vi "Cache-Kill.vi"(8 "error in":errorcluster, 11 "Idx":i32) -> (0 "error out":errorcluster)   [LabVIEW 2016]
uses:
  Cache.Action.ctl
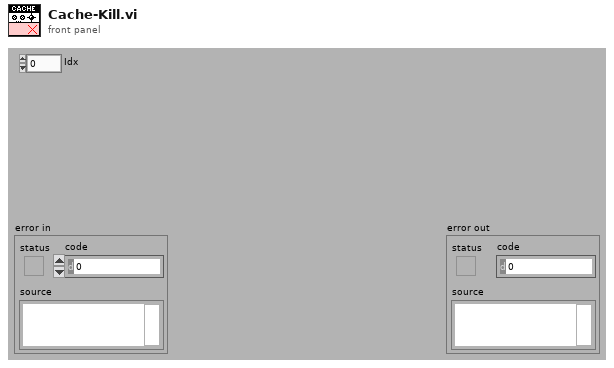
[diagram p1: front panel]
types:
  T1 = typedef "Cache.Action.ctl" = enum32{"idle", "constructor", "destructor", "--- Cache ---", "Find", "FindToExport", "Move", "Delete"}
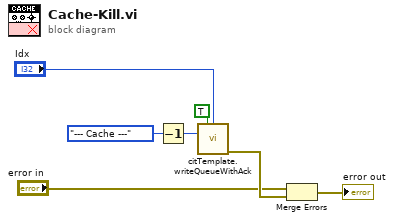
[diagram p0: block diagram]
diagram:
  n1 = Decrement(x=Cache.Action."--- Cache ---" ("Action")) -> (x-1=w4:T1)
  n2 = call "citTemplate.writeQueueWithAck.vi"("High priority (F)"=TRUE, "instance (0)"="Idx", "event in"=w4) -> ("error out"=w7:errorcluster)  [unwired: 10 in, 2 out]
  n3 = Merge Errors("error in", w7) -> (→"error out":errorcluster)
